vi "Example - How to use Nodes for Writing Test Bench.vi"() -> ()   [LabVIEW 2011]
panel:
  out "Channel Data":i16
  out "Sim IO FPGA Status":bool
  in  "Trig Data":bool
  in  "stop":bool
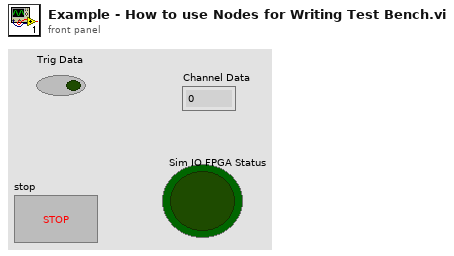
[diagram p1: front panel]
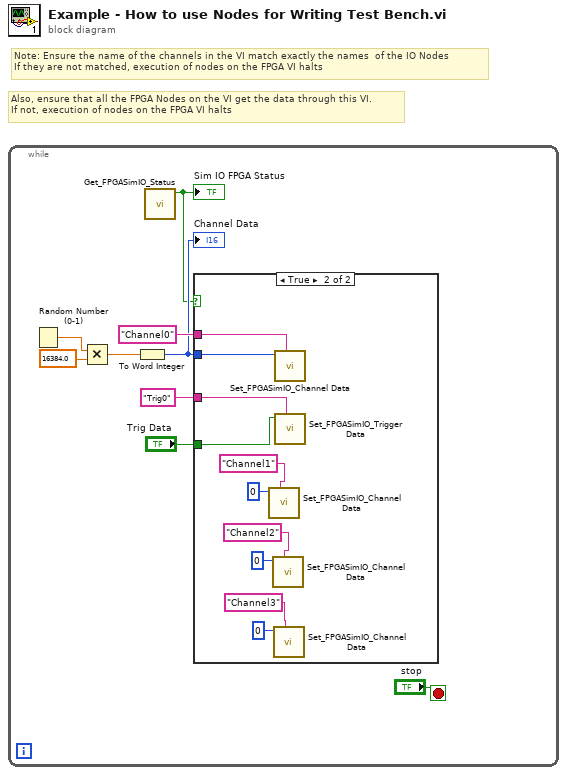
[diagram p0: block diagram]
diagram:
  # "Also, ensure that all the FPGA Nodes on the VI get the data through this VI.\nIf not, execution of nodes on the FPGA VI halts"
  # "Note: Ensure the name of the channels in the VI match exactly the names  of the IO Nodes\nIf they are not matched, execution of nodes on the FPGA VI halts"
  n1 = while {
    stop <- "stop" stop-if-true
    n2 = Random Number (0-1)() -> (number: 0 to 1=w5:dbl)
    n3 = Multiply(x=w5, y=16384.0) -> (x*y=w3:dbl)
    n4 = To Word Integer(number=w3) -> (16bit integer=w2:i16)
    "Channel Data" <- w2
    n5 = call <userlib>:"Get_FPGASimIO_Status.vi"() -> ("Sim IO FPGA Status"=w1:bool)  [unwired: 10 in, 1 out]
    "Sim IO FPGA Status" <- w1
    n6 = case shown="True" w1 {
      tunnel: "Channel0" ("IO Node Name") -> [_ w19]
      tunnel: "Trig0" ("IO Node Name") -> [_ w18]
      tunnel: "Trig Data" -> [_ w17]
      tunnel: w2 -> [_ w16]
      frame False {
      }
      frame True {
        n7 = call <userlib>:"Set_FPGASimIO_Channel Data.vi"("Channel Name"="Channel1" ("IO Node Name"), "Data"=i16 0) -> ()  [unwired: 9 in, 1 out]
        n8 = call <userlib>:"Set_FPGASimIO_Channel Data.vi"("Channel Name"="Channel2" ("IO Node Name"), "Data"=i16 0) -> ()  [unwired: 9 in, 1 out]
        n9 = call <userlib>:"Set_FPGASimIO_Channel Data.vi"("Channel Name"="Channel3" ("IO Node Name"), "Data"=i16 0) -> ()  [unwired: 9 in, 1 out]
        n10 = call <userlib>:"Set_FPGASimIO_Channel Data.vi"("Channel Name"=w19, "Data"=w16) -> ()  [unwired: 9 in, 1 out]
        n11 = call <userlib>:"Set_FPGASimIO_Trigger Data.vi"("Channel Name"=w18, "Trig Data"=w17) -> ()  [unwired: 9 in, 1 out]
      }
    }
  }
